vi "Generate Signal.vi"(8 "error in (no error)":errorcluster, 9 "Amplitude (1)":dbl=0.5, 10 "Frequency (1000 Hz)":dbl=1000.0, 11 "NI Sig Gen in":refnum<class "NI Sig Gen.lvclass">) -> (0 "error out":errorcluster, 3 "NI Sig Gen out":refnum<class "NI Sig Gen.lvclass">)   [LabVIEW 2010, in "NI Sig Gen.lvclass"]
uses:
  NI Sig Gen.lvclass
  <instrlib>/niFgen/niFgen.llb/niFgen Waveform Type.ctl
  NI Sig Gen.lvclass/NI Sig Gen.ctl
panel:
  in  "Waveform":T1 items=["Sine", "Square", "Triangle", "Ramp Up", "Ramp Down", "DC", "Noise", "User"]
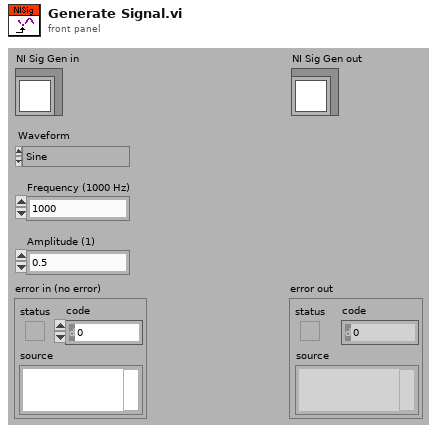
[diagram p1: front panel]
types:
  T1 = typedef "niFgen Waveform Type.ctl" = i32
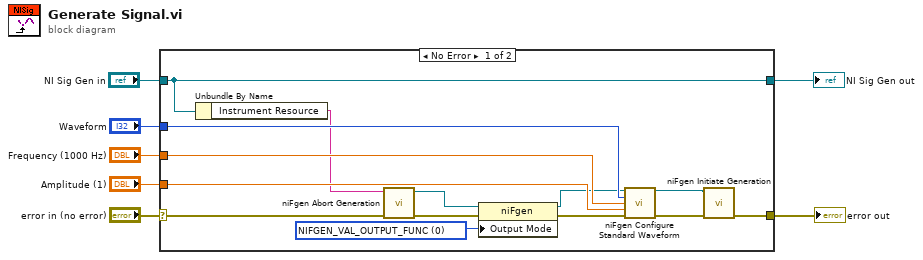
[diagram p0: block diagram]
diagram:
  n1 = case shown="No Error" "error in (no error)" {
    selector: "error in (no error)" -> [w10 w23]
    tunnel: [w17 w23] -> w4
    tunnel: "Amplitude (1)" -> [w18 _]
    tunnel: "Frequency (1000 Hz)" -> [w19 _]
    tunnel: "Waveform" -> [w16 _]
    tunnel: "NI Sig Gen in" -> [w9 w22]
    tunnel: [w9 w22] -> w1
    frame No Error {
      w15 = 0 items=["NIFGEN_VAL_OUTPUT_FUNC"=0, "NIFGEN_VAL_OUTPUT_FREQ_LIST"=101, "NIFGEN_VAL_OUTPUT_ARB"=1, "NIFGEN_VAL_OUTPUT_SEQ"=2, "NIFGEN_VAL_OUTPUT_SCRIPT"=102] ("Basic Operation:Output Mode")
      n2 = Unbundle By Name(w9) -> ("Instrument Resource"=w8:string)
      n3 = call <instrlib>:"niFgen Abort Generation.vi"("error in (no error)"=w10, "Instrument Handle"=w8) -> ("error out"=w12:errorcluster, "Instrument Handle Out"=w11:refnum<k15>)  [unwired: 8 out]
      n4 = property class="niFgen"(reference=w11, error in=w12, "Output Mode"=w15) -> (reference out=w13:refnum<k15>, error out=w14:errorcluster)
      n5 = call <instrlib>:"niFgen Configure Standard Waveform.vi"("Instrument Handle"=w13, "Waveform"=w16, "Frequency"=w19, "Amplitude"=w18, "error in (no error)"=w14) -> ("Instrument Handle Out"=w20:refnum<k15>, "error out"=w21:errorcluster)  [unwired: 3 in, 6 out]
      n6 = call <instrlib>:"niFgen Initiate Generation.vi"("error in (no error)"=w21, "Instrument Handle"=w20) -> ("error out"=w17:errorcluster)  [unwired: 9 out]
    }
    frame Error {
    }
  }
  "error out" <- w4
  "NI Sig Gen out" <- w1
